vi "Drive Forward to Position.vi"(5 "output rate (EGU/min)":dbl=1.0 format="%.2f", 6 "PID gains":T1={"proportional gain (Kc)"=0.001, "integral time (Ti, min)"=0.0, "derivative time (Td, min)"=0.0} {"derivative time (Td, min)" format="%.3f"; "integral time (Ti, min)" format="%.3f"; "proportional gain (Kc)" format="%.3f"}, 7 "output range":cluster{"output high":dbl, "output low":dbl}={"output high"=0.8, "output low"=-0.8}, 8 "error in (no error)":errorcluster, 9 "Speed":dbl=0.5, 10 "Target":dbl=158.0 format="%#_13g", 11 "AutonRef":T2={"Starting Pos"=0, "Defence"=enum."Low Bar", "Drivetrain"={"DevStatus"={"status"=FALSE, "code"=0, "source"=""}, "Motors[]"=[{"DeviceStatus"={"status"=FALSE, "code"=0, "source"=""}, "Type"=enum."PWM", "PWM"={"PWM Channel"=enum."PWM 0", "DeadBand"={"Name"="SPARK", "maxPositivePwm"=1500, "minPositivePwm"=1010, "centerPwm"=1005, "maxNegativePwm"=1000, "minNegativePwm"=500, "angularRange"=0}}, "CAN"={"Device Number"=0, "Control Mode"=enum."Percent VBus", "Semaphore"=refnum, "Max Vout"=0.0, "TalonSRX Control Mode"=enum."Percent VBus"}, "Invert"=FALSE}, {"DeviceStatus"={"status"=FALSE, "code"=0, "source"=""}, "Type"=enum."PWM", "PWM"={"PWM Channel"=enum."PWM 1", "DeadBand"={"Name"="SPARK", "maxPositivePwm"=1500, "minPositivePwm"=1010, "centerPwm"=1005, "maxNegativePwm"=1000, "minNegativePwm"=500, "angularRange"=0}}, "CAN"={"Device Number"=0, "Control Mode"=enum."Percent VBus", "Semaphore"=refnum, "Max Vout"=0.0, "TalonSRX Control Mode"=enum."Percent VBus"}, "Invert"=TRUE}], "Square Inputs"=TRUE, "Max Output"=1.0}, "State"=enum."Drive to Outerworks", "Encoder Right"={"DevStatus"={"status"=FALSE, "code"=0, "source"=""}, "EncoderIndex"=enum."Enc 1", "CounterIndex"=enum."Invalid", "DistancePerCount"=0.008181230868723419, "Decoding Type"=enum."4x"}, "Encoder Left"={"DevStatus"={"status"=FALSE, "code"=0, "source"=""}, "EncoderIndex"=enum."Enc 0", "CounterIndex"=enum."Invalid", "DistancePerCount"=0.008181230868723419, "Decoding Type"=enum."4x"}, "Line Sensor"={"DevStatus"={"status"=FALSE, "code"=0, "source"=""}, "DIO Channel"=enum."DIO 9", "CntIndex"=enum."Invalid", "Normally Closed"=FALSE}, "navX"={"Interface"={"Protocol"=enum."SPI", "Update Rate (4Hz-60Hz)"=50, "navX Open TypeDef"=variant(cluster{"SPI Bus":enum16{"SPI On-Board, CS0", "SPI On-Board, CS1", "SPI On-Board, CS2", "SPI On-Board, CS3", "SPI MXP", "Invalid"}, "Clock Rate (Hz)":dbl} {"SPI Bus"=enum."SPI On-Board, CS0", "Clock Rate (Hz)"=2000000.0})}, "Notify Packet"=refnum, "Loop VI Refnum"=refnum, "Ready to Close Occurrence Refnum"=refnum}, "Front Arm"={"DevStatus"={"status"=FALSE, "code"=0, "source"=""}, "Analog Channel"=enum."Invalid", "Invert Output"=FALSE}, "Start Time"=0, "State Vars"=variant} {"navX"."Interface"."Update Rate (4Hz-60Hz)" min=4 max=60 step=1}) -> (0 "error out":errorcluster, 2 "Encoder Difference":dbl=9.15275203438432, 3 "Angle Error":dbl=0.004439899999999999)   [LabVIEW 2015]
uses:
  Typedef/AutonRefType.ctl
  Typedef/Defences.ctl
  <vilib>/Rock Robotics/WPI/RobotDrive/WPI_RobotDriveDevRef.ctl
  <vilib>/Rock Robotics/WPI/MotorControl/WPI_MotorControlDeviceRef.ctl
  <vilib>/Rock Robotics/WPI/MotorControl/WPI_MotorControlType.ctl
  <vilib>/Rock Robotics/SystemInterfaces/DIO/FPGA_DIOPWMChannel.ctl
  <vilib>/Rock Robotics/WPI/PWM/WPI_PWMDeadband.ctl
  <vilib>/Rock Robotics/WPI/CAN/Jaguar/SubVIs/WPI_CANJaguar_ControlMode.ctl
  <vilib>/Rock Robotics/WPI/CAN/TalonSRX/WPI_CANTalonSRX_APIControlMode.ctl
  Typedef/MainStates.ctl
  <vilib>/Rock Robotics/WPI/Encoder/WPI_EncoderDevRef.ctl
  <vilib>/Rock Robotics/SystemInterfaces/Encoder/FPGA_EncoderIdx.ctl
  <vilib>/Rock Robotics/SystemInterfaces/Counter/FPGA_CounterCtrSystemIndex.ctl
  <vilib>/Rock Robotics/WPI/Encoder/WPI_EncoderType.ctl
  <vilib>/Rock Robotics/WPI/Switch/WPI_SwitchDevRef.ctl
  <vilib>/Rock Robotics/SystemInterfaces/DIO/FPGA_DIOChannel.ctl
  NavX/TypeDefs/Z900_navX_DeviceTypeDef.ctl
  NavX/TypeDefs/Z900_navX_ProtocolTypeDef.ctl
  NavX/TypeDefs/Z900_navX_NotifyPacketTypeDef.ctl
  NavX/TypeDefs/Z900_navX_ActionTypeDef.ctl
  <vilib>/Rock Robotics/WPI/Potentiometer/WPI_PotentiometerDevRef.ctl
  <vilib>/Rock Robotics/SystemInterfaces/AI/FPGA_AIChannel.ctl
  <vilib>/addons/control/pid/pid.llb/PID (DBL).vi
  <vilib>/Rock Robotics/WPI/RobotDrive/WPI_RobotDriveArcadeDrive_RatioCurve.vi
  <vilib>/addons/control/pid/pid.llb/PID Output Rate Limiter (DBL).vi
  <vilib>/addons/control/pid/NI_PID_pid.lvlib
  NavX/navX Library v2.lvlib
  <vilib>/ptbypt/NI_PtbyPt.lvlib
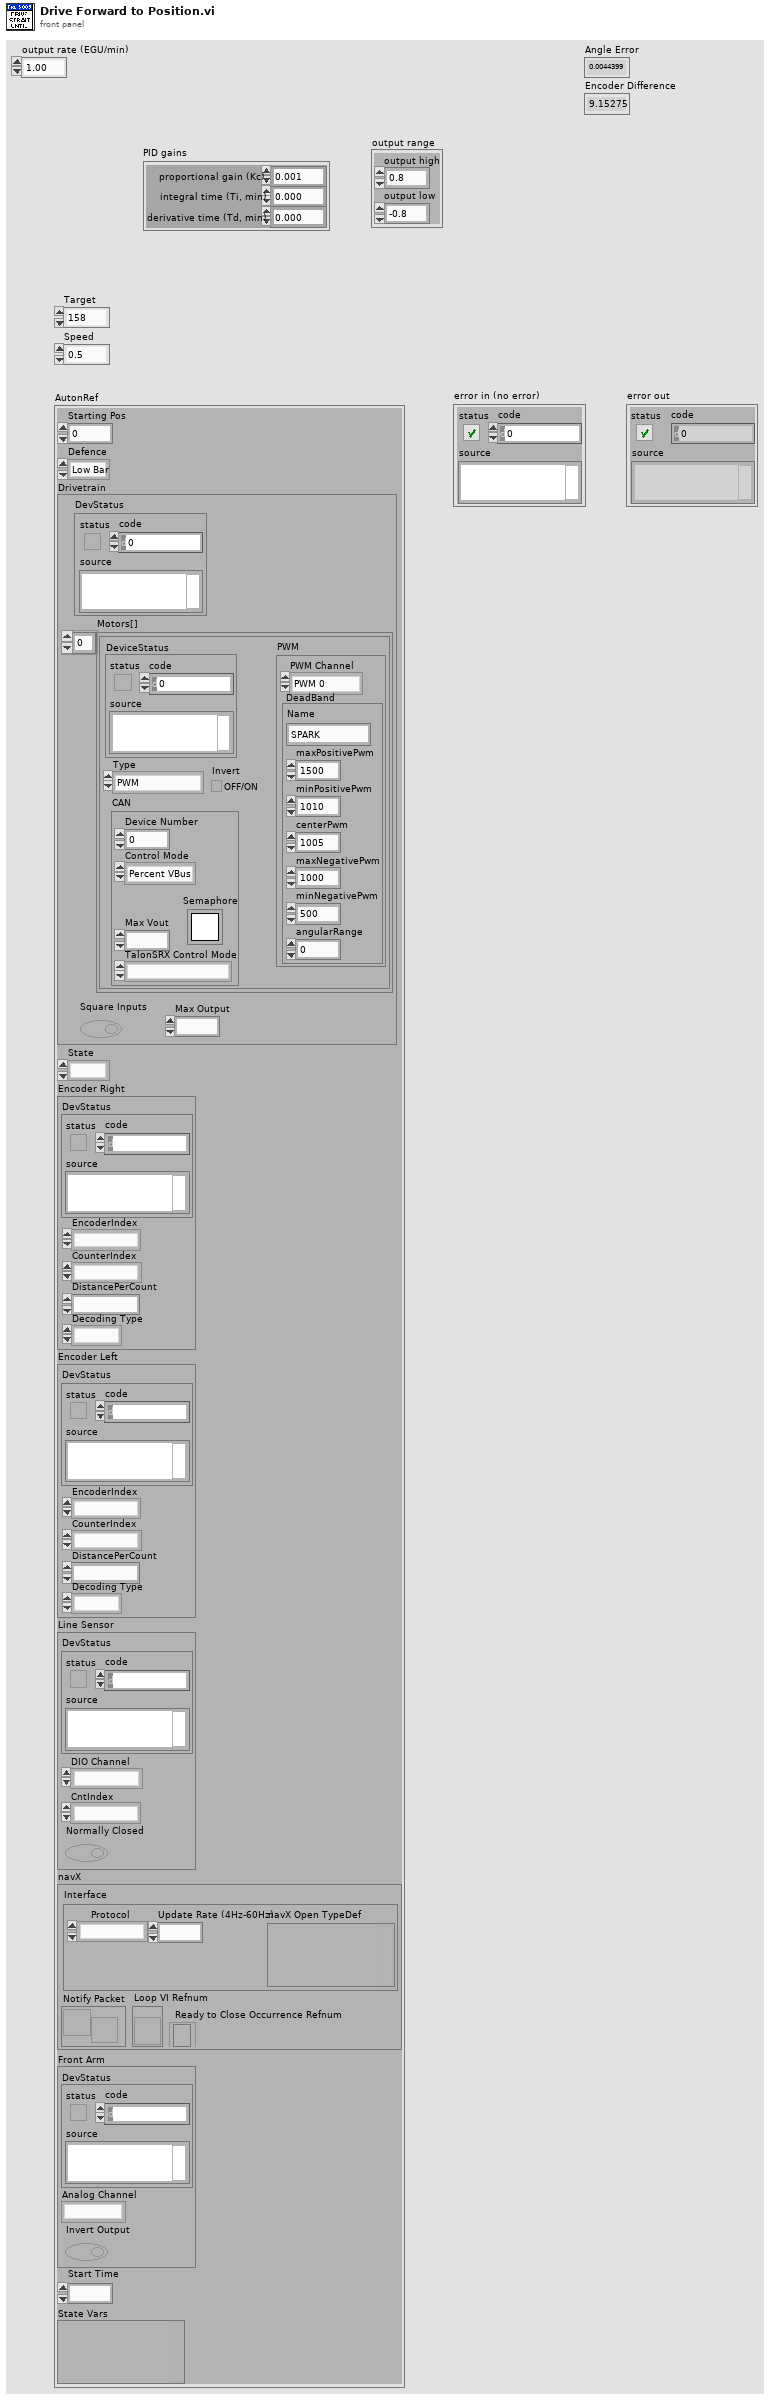
[diagram p1: front panel]
types:
  T1 = cluster{"proportional gain (Kc)":dbl, "integral time (Ti, min)":dbl, "derivative time (Td, min)":dbl}
  T2 = typedef "AutonRefType.ctl" = cluster{"Starting Pos":u32, "Defence":T3, "Drivetrain":T4, "State":T12, "Encoder Right":T13, "Encoder Left":T13, "Line Sensor":T17, "navX":T19, "Front Arm":T21, "Start Time":u32, "State Vars":variant}
  T3 = typedef "Defences.ctl" = enum16{"Low Bar", "Chivel De Fris", "Sally Port", "Portcullis", "Draw Bridge", "Moat", "Rough Terrain", "Ramparts", "Rock Wall"}
  T4 = typedef "WPI_RobotDriveDevRef.ctl" = cluster{"DevStatus":errorcluster, "Motors[]":T5[], "Square Inputs":bool, "Max Output":dbl}
  T5 = typedef "WPI_MotorControlDeviceRef.ctl" = cluster{"DeviceStatus":errorcluster, "Type":T6, "PWM":cluster{"PWM Channel":T7, "DeadBand":T8}, "CAN":cluster{"Device Number":u8, "Control Mode":T9, "Semaphore":T10, "Max Vout":dbl, "TalonSRX Control Mode":T11}, "Invert":bool}
  T6 = typedef "WPI_MotorControlType.ctl" = enum16{"PWM", "CAN", "CANTalonSRX"}
  T7 = typedef "FPGA_DIOPWMChannel.ctl" = enum8{"PWM 0", "PWM 1", "PWM 2", "PWM 3", "PWM 4", "PWM 5", "PWM 6", "PWM 7", "PWM 8", "PWM 9", "PWM MXP 0", "PWM MXP 1", "PWM MXP 2", "PWM MXP 3", "PWM MXP 4", "PWM MXP 5", "PWM MXP 6", "PWM MXP 7", "PWM MXP 8", "PWM MXP 9", "Invalid"}
  T8 = typedef "WPI_PWMDeadband.ctl" = cluster{"Name":string, "maxPositivePwm":i32, "minPositivePwm":i32, "centerPwm":i32, "maxNegativePwm":i32, "minNegativePwm":i32, "angularRange":u16}
  T9 = typedef "WPI_CANJaguar_ControlMode.ctl" = enum8{"Percent VBus", "Current", "Speed", "Position", "Voltage"}
  T10 = typedef "Semaphore RefNum" = refnum<k1>
  T11 = typedef "WPI_CANTalonSRX_APIControlMode.ctl" = enum8{"Percent VBus", "Speed", "Position", "Slave", "Unchanged / Invalid", "Voltage Compensation", "Current", "Motion Profile"}
  T12 = typedef "MainStates.ctl" = enum16{"Drive to Outerworks", "Cross Defence", "Align to Line", "Turn to Goal", "Find Position", "Find Distance", "Drive to Scoring Location", "Score Low Goal", "SquareToField", "Hit Driver Station Wall", "Drive Back to Position", "CDF", "Cleanup", "_TEST_Profile", "_TEST_TurnProfile", "_TEST_Impulse", "Error"}
  T13 = typedef "WPI_EncoderDevRef.ctl" = cluster{"DevStatus":errorcluster, "EncoderIndex":T14, "CounterIndex":T15, "DistancePerCount":dbl, "Decoding Type":T16}
  T14 = typedef "FPGA_EncoderIdx.ctl" = enum8{"Enc 0", "Enc 1", "Enc 2", "Enc 3", "Enc 4", "Enc 5", "Enc 6", "Enc 7", "Invalid"}
  T15 = typedef "FPGA_CounterCtrSystemIndex.ctl" = enum8{"Ctr 0", "Ctr 1", "Ctr 2", "Ctr 3", "Ctr 4", "Ctr 5", "Ctr 6", "Ctr 7", "Invalid"}
  T16 = typedef "WPI_EncoderType.ctl" = enum16{"1x", "2x", "4x"}
  T17 = typedef "WPI_SwitchDevRef.ctl" = cluster{"DevStatus":errorcluster, "DIO Channel":T18, "CntIndex":T15, "Normally Closed":bool}
  T18 = typedef "FPGA_DIOChannel.ctl" = enum8{"DIO 0", "DIO 1", "DIO 2", "DIO 3", "DIO 4", "DIO 5", "DIO 6", "DIO 7", "DIO 8", "DIO 9", "DIO MXP 0", "DIO MXP 1", "DIO MXP 2", "DIO MXP 3", "DIO MXP 4", "DIO MXP 5", "DIO MXP 6", "DIO MXP 7", "DIO MXP 8", "DIO MXP 9", "DIO MXP 10", "DIO MXP 11", "DIO MXP 12", "DIO MXP 13", "DIO MXP 14", "DIO MXP 15", "Invalid"}
  T19 = typedef "navX Library v2.lvlib/Z900_navX_DeviceTypeDef.ctl" = cluster{"Interface":cluster{"Protocol":T20, "Update Rate (4Hz-60Hz)":u8, "navX Open TypeDef":variant}, "Notify Packet":refnum<notifier>, "Loop VI Refnum":refnum<vi>, "Ready to Close Occurrence Refnum":refnum<k4>}
  T20 = typedef "navX Library v2.lvlib/Z900_navX_ProtocolTypeDef.ctl" = enum16{"SERIAL", "I2C", "SPI"}
  T21 = typedef "WPI_PotentiometerDevRef.ctl" = cluster{"DevStatus":errorcluster, "Analog Channel":T22, "Invert Output":bool}
  T22 = typedef "FPGA_AIChannel.ctl" = enum8{"AI 0", "AI 1", "AI 2", "AI 3", "AI MXP 0", "AI MXP 1", "AI MXP 2", "AI MXP 3", "Invalid"}
  T23 = cluster{"Yaw":dbl, "Roll":dbl, "Pitch":dbl, "Heading":dbl, "Fused Heading":dbl}
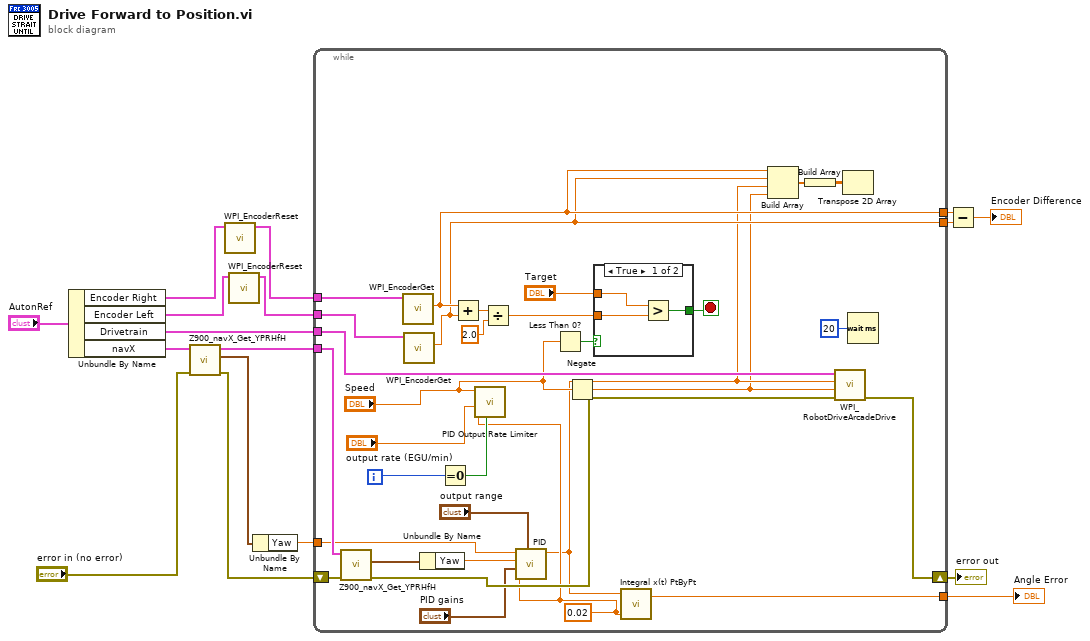
[diagram p0: block diagram]
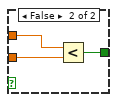
[diagram p2: hidden frame]
diagram:
  n1 = Unbundle By Name("AutonRef") -> ("Encoder Right"=w4:T13, "Encoder Left"=w2:T13, "Drivetrain"=w17:T4, "navX"=w13:T19)
  n2 = call "Z900_navX_Get_YPRHfH.vi"("error in (no error)"="error in (no error)", "navX Device"=w13) -> ("error out"=w10:errorcluster, "YRPHfH"=w15:T23, "navX Device"=w12:T19)  [unwired: 6 in, 1 out]
  n3 = call <vilib>:"WPI_EncoderReset.vi"("EncoderDevRef"=w4) -> ("EncoderDevRef"=w3:T13)  [unwired: 9 in, 1 out]
  n4 = call <vilib>:"WPI_EncoderReset.vi"("EncoderDevRef"=w2) -> ("EncoderDevRef"=w1:T13)  [unwired: 9 in, 1 out]
  n5 = Unbundle By Name(w15) -> ("Yaw"=w14:dbl)
  n6 = while {
    tunnel: w3 -> [w48]
    tunnel: w1 -> [w47]
    tunnel: w17 -> [w46]
    tunnel: [w32] -> w8
    tunnel: w14 -> [w42]
    tunnel: w12 -> [w43]
    shift-right: [w33] -> w9
    shift-left: w10 -> [w35]
    tunnel: [w23] -> w6
    tunnel: [w22] -> w7
    i -> [w27]
    stop <- w36 stop-if-true
    w26 = 0.02 ("dt")
    n7 = call "Z900_navX_Get_YPRHfH.vi"("error in (no error)"=w35, "navX Device"=w43) -> ("error out"=w34:errorcluster, "YRPHfH"=w45:T23)  [unwired: 6 in, 2 out]
    n8 = call <vilib>:"WPI_EncoderGet.vi"("EncoderDevRef"=w48) -> ("Distance"=w23:dbl)  [unwired: 5 in, 5 out]
    n9 = call <vilib>:"WPI_EncoderGet.vi"("EncoderDevRef"=w47) -> ("Distance"=w22:dbl)  [unwired: 5 in, 5 out]
    n10 = Unbundle By Name(w45) -> ("Yaw"=w44:dbl)
    n11 = Equal To 0?(x=w27) -> (x = 0?=w28:bool)
    n12 = Add(x=w23, y=w22) -> (x+y=w41:dbl)
    n13 = call-poly <vilib>:"PID Output Rate Limiter.vi"("reinitialize? (F)"=w28, "dt (s)"=w26, "output rate (EGU/min)"="output rate (EGU/min)", "input (controller output)"="Speed") -> ()  [unwired: 4 in, 2 out]
    n14 = Divide(x=w41, y=2.0) -> (x/y=w38:dbl)
    n15 = call-poly <vilib>:"PID.vi"("output range"="output range", "dt (s)"=w26, "PID gains"="PID gains", "process variable"=w44, "setpoint"=w42) -> ("output"=w19:dbl)  [unwired: 5 in, 1 out]
    n16 = Less Than 0?(x="Speed") -> (x < 0?=w39:bool)
    n17 = Negate(x="Speed") -> (-x=w18:dbl)
    n18 = case shown="True" w39 {
      tunnel: w38 -> [w50 w53]
      tunnel: "Target" -> [w51 w54]
      tunnel: [w49 w52] -> w36
      frame True {
        n19 = Greater?(x=w51, y=w50) -> (0:w49:bool)
      }
      frame False {
        n20 = Less?(x=w54, y=w53) -> (x < y?=w52:bool)
      }
    }
    n21 = call <vilib>:"Integral x(t) PtByPt.vi"("dt"=w26, "x"=w19) -> ("integral x(t)"=w32:dbl)  [unwired: 2 in, 1 out]
    n22 = Build Array(w23, w22, w19, w18) -> (w21:dbl[])
    n23 = Build Array(w21) -> (w20:dbl[][])
    n24 = call-poly <vilib>:"WPI_RobotDriveArcadeDrive.vi"("error in (no error)"=w34, "Y axis value (Speed)"=w18, "X axis value (Curve)"=w19, "RobotDriveDevRef"=w46) -> ("error out"=w33:errorcluster)  [unwired: 5 in, 2 out]
    n25 = Transpose 2D Array(2D array=w20) -> ()  [unwired: 1 out]
    n26 = Wait (ms)(milliseconds to wait=u32 20) -> ()  [unwired: 1 out]
  }
  "error out" <- w9
  "Angle Error" <- w8
  n27 = Subtract(x=w6, y=w7) -> (x-y=→"Encoder Difference":dbl)
